vi "VCS Get Ssi Abs Encoder ParameterEx.vi"(6 "error in (no error)":errorcluster, 9 "axis in":cluster{"keyHandle":u32, "nodeId":u16}={"keyHandle"=0, "nodeId"=1}) -> (0 "error out":errorcluster, 1 "SSI encoder":T1, 3 "axis out":cluster{"keyHandle":u32, "nodeId":u16}={"keyHandle"=0, "nodeId"=1})   [LabVIEW 2010]
doc: "With function <B>VCS_GetSsiAbsEncoderParameter</B> it is possible to read all parameters from SSI absolute encoder."
uses:
  Resources/EposCmd.dll
  Resources/EposCmd64.dll
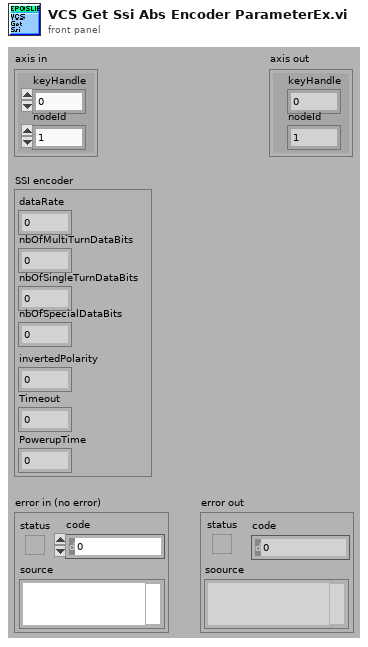
[diagram p1: front panel]
types:
  T1 = cluster{"dataRate":u16, "nbOfMultiTurnDataBits":u16, "nbOfSingleTurnDataBits":u16, "nbOfSpecialDataBits":u16, "invertedPolarity":i32, "Timeout":u16, "PowerupTime":u16}
  T2 = cluster{"pDataRate":u16, "pNbOfMultiTurnDataBits":u16, "pNbOfSingleTurnDataBits":u16, "pNbOfSpecialDataBits":u16, "pInvertedPolarity":i32, "pTimeout":u16, "pPowerupTime":u16}
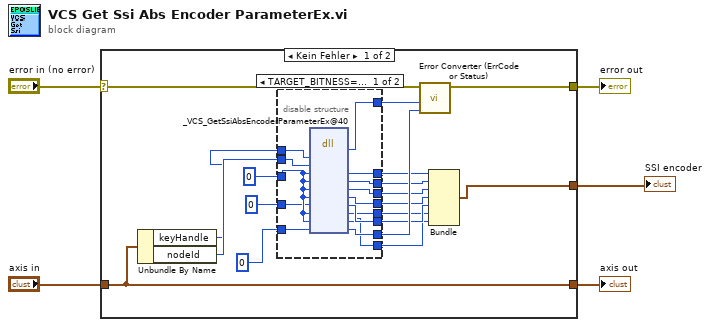
[diagram p0: block diagram]
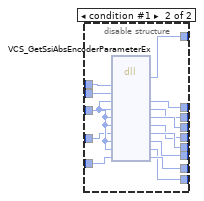
[diagram p2: hidden frame]
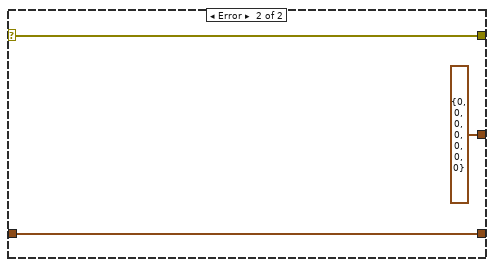
[diagram p3: hidden frame]
diagram:
  n1 = case shown="Kein Fehler" "error in (no error)" {
    selector: "error in (no error)" -> [w21 w53]
    tunnel: "axis in" -> [w23 w54]
    tunnel: [w23 w54] -> w4
    tunnel: [w22 w53] -> w3
    tunnel: [w6 T2 {"pDataRate"=0, "pNbOfMultiTurnDataBits"=0, "pNbOfSingleTurnDataBits"=0, "pNbOfSpecialDataBits"=0, "pInvertedPolarity"=0, "pTimeout"=0, "pPowerupTime"=0}] -> w1
    frame No Error {
      n2 = Unbundle By Name(w23) -> ("keyHandle"=w16:u32, "nodeId"=w17:u16)
      n3 = disable-structure shown="TARGET_BITNESS==32, Standard" {
        disable-tunnel: [w32 w51] -> w20
        disable-tunnel: [w31 w50] -> w19
        disable-tunnel: u32 0 ("pErrorCode") -> [w34 w49]
        disable-tunnel: w17 -> [w36 w48]
        disable-tunnel: w16 -> [w37 w47]
        disable-tunnel: u16 0 ("pDataRate") -> [w35 w46]
        disable-tunnel: 0 ("pInvertedPolarity") -> [w33 w45]
        disable-tunnel: [w30 w38] -> w13
        disable-tunnel: [w29 w39] -> w12
        disable-tunnel: [w28 w40] -> w11
        disable-tunnel: [w27 w41] -> w10
        disable-tunnel: [w26 w43] -> w9
        disable-tunnel: [w25 w42] -> w8
        disable-tunnel: [w24 w44] -> w7
        frame condition #0 (active) {
          n4 = dll-call lib="C:/Sources/LabVIEW/maxon EPOS/Resources/EposCmd.*" fn="_VCS_GetSsiAbsEncoderParameterEx@40" ("EposCmd.dll:_VCS_GetSsiAbsEncoderParameter@28")("KeyHandle"=w37, "NodeId"=w36, "pDataRate"=w35, "pNbOfMultiTurnDataBits"=w35, "pNbOfSingleTurnDataBits"=w35, "pNbOfSpecialDataBits"=w35, "pInvertedPolarity"=w33, "pTimeout"=w35, "pPowerupTime"=w35, "pErrorCode"=w34) -> ("Rückgabetyp"=w31:i32, "pDataRate"=w30:u16, "pNbOfMultiTurnDataBits"=w29:u16, "pNbOfSingleTurnDataBits"=w28:u16, "pNbOfSpecialDataBits"=w27:u16, "pInvertedPolarity"=w26:i32, "pTimeout"=w25:u16, "pPowerupTime"=w24:u16, "pErrorCode"=w32:u32)  [unwired: 5 in, 2 out]
        }
        frame condition #1 {
          n5 = dll-call lib="C:/Sources/LabVIEW/maxon EPOS/Resources/EposCmd64.dll" fn="VCS_GetSsiAbsEncoderParameterEx" ("EposCmd.dll:_VCS_GetSsiAbsEncoderParameter@28")("KeyHandle"=w47, "NodeId"=w48, "pDataRate"=w46, "pNbOfMultiTurnDataBits"=w46, "pNbOfSingleTurnDataBits"=w46, "pNbOfSpecialDataBits"=w46, "pInvertedPolarity"=w45, "pTimeout"=w46, "pPowerupTime"=w46, "pErrorCode"=w49) -> ("Rückgabetyp"=w50:i32, "pDataRate"=w38:u16, "pNbOfMultiTurnDataBits"=w39:u16, "pNbOfSingleTurnDataBits"=w40:u16, "pNbOfSpecialDataBits"=w41:u16, "pInvertedPolarity"=w42:i32, "pTimeout"=w43:u16, "pPowerupTime"=w44:u16, "pErrorCode"=w51:u32)  [unwired: 5 in, 2 out]
        }
      }
      n6 = call "Error Converter (ErrCode or Status).vi"("error code"=w20, "return type"=w19, "error in (no error)"=w21) -> ("error out"=w22:errorcluster)  [unwired: 7 in]
      n7 = Bundle("pDataRate"=w13, "pNbOfMultiTurnDataBits"=w12, "pNbOfSingleTurnDataBits"=w11, "pNbOfSpecialDataBits"=w10, "pInvertedPolarity"=w9, "pTimeout"=w8, "pPowerupTime"=w7) -> (w6:T2)  [unwired: 1 in]
    }
    frame Error {
    }
  }
  "error out" <- w3
  "axis out" <- w4
  "SSI encoder" <- w1
